vi "Set MeasurementService GetMetadata Response.vi"(7 "Streaming? (F)":bool, 8 "error in (no error)":errorcluster, 10 "Message Data":T1, 11 "gRPCid in":T10) -> (0 "error out":errorcluster)   [LabVIEW 2020, in "MeasurementLink Measurement Service V2.lvlib" / "MeasurementService.lvclass"]
uses:
  MeasurementService.lvclass
  <vilib>/gRPC/LabVIEW gRPC Library/Shared/grpcId.ctl
  RPC Messages/ni_measurementlink_measurement_v2_GetMetadataResponse.ctl
  RPC Messages/ni_measurementlink_measurement_v2_MeasurementDetails.ctl
  RPC Messages/ni_measurementlink_measurement_v2_MeasurementSignature.ctl
  RPC Messages/ni_measurementlink_measurement_v2_ConfigurationParameter.ctl
  RPC Messages/ni_measurementlink_measurement_v2_ConfigurationParameter_AnnotationsEntry.ctl
  RPC Messages/google_protobuf_Any.ctl
  RPC Messages/ni_measurementlink_measurement_v2_Output.ctl
  RPC Messages/ni_measurementlink_measurement_v2_Output_AnnotationsEntry.ctl
  RPC Messages/ni_measurementlink_measurement_v2_UserInterfaceDetails.ctl
  MeasurementLink Measurement Service V2.lvlib
  <vilib>/gRPC/LabVIEW gRPC Library/grpc-lvsupport-release.lvlib
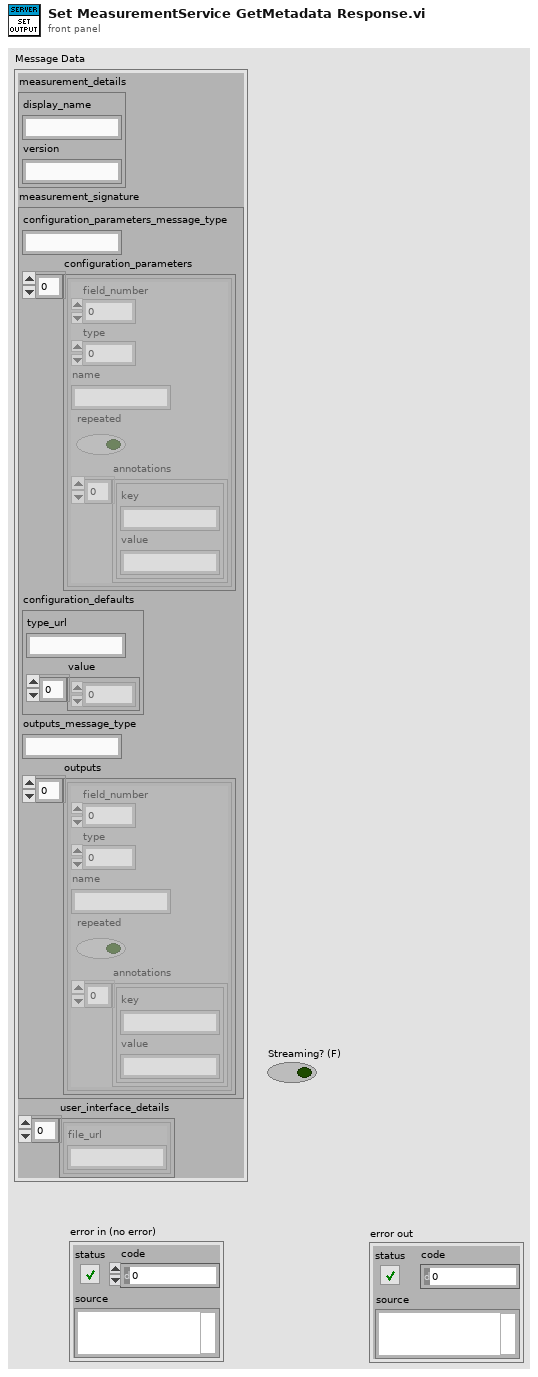
[diagram p1: front panel]
types:
  T1 = typedef "MeasurementLink Measurement Service V2.lvlib/ni_measurementlink_measurement_v2_GetMetadataResponse.ctl" = cluster{"measurement_details":T2, "measurement_signature":T3, "user_interface_details":T9[]}
  T2 = typedef "MeasurementLink Measurement Service V2.lvlib/ni_measurementlink_measurement_v2_MeasurementDetails.ctl" = cluster{"display_name":string, "version":string}
  T3 = typedef "MeasurementLink Measurement Service V2.lvlib/ni_measurementlink_measurement_v2_MeasurementSignature.ctl" = cluster{"configuration_parameters_message_type":string, "configuration_parameters":T4[], "configuration_defaults":T6, "outputs_message_type":string, "outputs":T7[]}
  T4 = typedef "MeasurementLink Measurement Service V2.lvlib/ni_measurementlink_measurement_v2_ConfigurationParameter.ctl" = cluster{"field_number":i32, "type":i32, "name":string, "repeated":bool, "annotations":T5[]}
  T5 = typedef "MeasurementLink Measurement Service V2.lvlib/ni_measurementlink_measurement_v2_ConfigurationParameter_AnnotationsEntry.ctl" = cluster{"key":string, "value":string}
  T6 = typedef "MeasurementLink Measurement Service V2.lvlib/google_protobuf_Any.ctl" = cluster{"type_url":string, "value":u8[]}
  T7 = typedef "MeasurementLink Measurement Service V2.lvlib/ni_measurementlink_measurement_v2_Output.ctl" = cluster{"field_number":i32, "type":i32, "name":string, "repeated":bool, "annotations":T8[]}
  T8 = typedef "MeasurementLink Measurement Service V2.lvlib/ni_measurementlink_measurement_v2_Output_AnnotationsEntry.ctl" = cluster{"key":string, "value":string}
  T9 = typedef "MeasurementLink Measurement Service V2.lvlib/ni_measurementlink_measurement_v2_UserInterfaceDetails.ctl" = cluster{"file_url":string}
  T10 = typedef "grpc-lvsupport-release.lvlib/grpcId.ctl" = u64
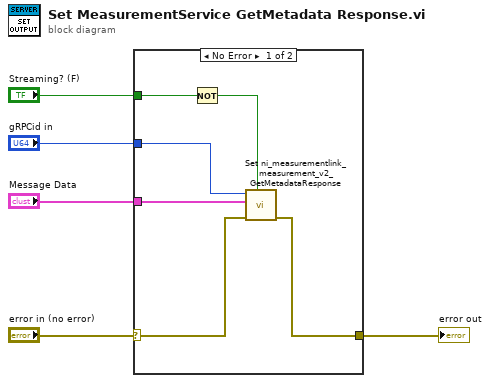
[diagram p0: block diagram]
diagram:
  n1 = case shown="No Error" "error in (no error)" {
    selector: "error in (no error)" -> [w11 w12]
    tunnel: [w9 w12] -> w4
    tunnel: "gRPCid in" -> [w10 _]
    tunnel: "Message Data" -> [w8 _]
    tunnel: "Streaming? (F)" -> [w7 _]
    frame No Error {
      n2 = Not(x=w7) -> (.not. x?=w6:bool)
      n3 = call "Set ni_measurementlink_measurement_v2_GetMetadataResponse.vi"("Complete Call (T)"=w6, "error in (no error)"=w11, "package_templatemessage"=w8, "gRPCid"=w10) -> ("error out"=w9:errorcluster)  [unwired: 7 in]
    }
    frame Error {
    }
  }
  "error out" <- w4
